vi "Client simulator.vi"() -> ()   [LabVIEW 2011]
panel:
  in  "?":bool
  in  "Port":u16=8222 min=1025 step=1
  out "FINAL FRAME":string[](array[string])
  out "CHECK SUM":u8=202 format="%01x"
  out "ANALOG PAR":u8[](array[numeric]) format="%02x"
  out "Array 2":bool[][](array[boolean])
  out "DIGITAL PAR":u8[](array[numeric]) format="%02x"
  in  "FT":string[](array[string])
  in  "stop":bool
  in  "Stop sync":string[](array[string])
  in  "Start sync":string[](array[string])
  in  "DCNT":string[](array[string])
  in  "ACNT":string[](array[string])
  in  "Digital parameters":i32(listbox)
  in  "Analog parameters":i32(listbox)
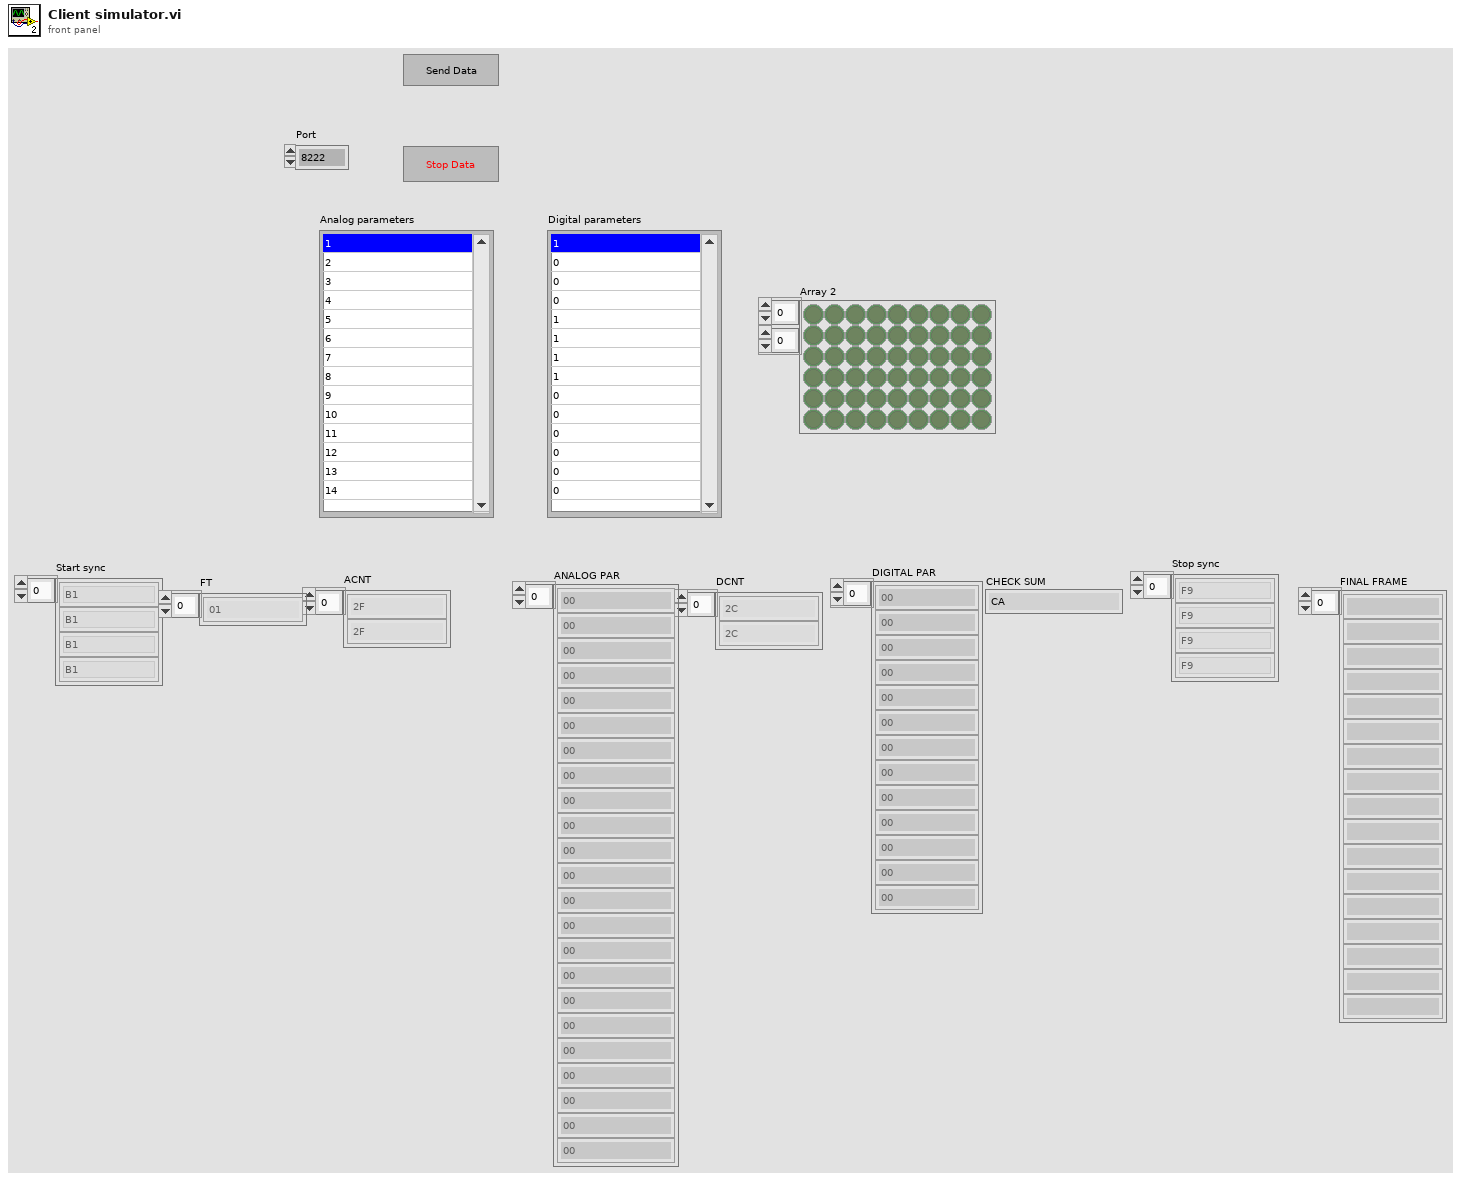
[diagram p1: front panel]
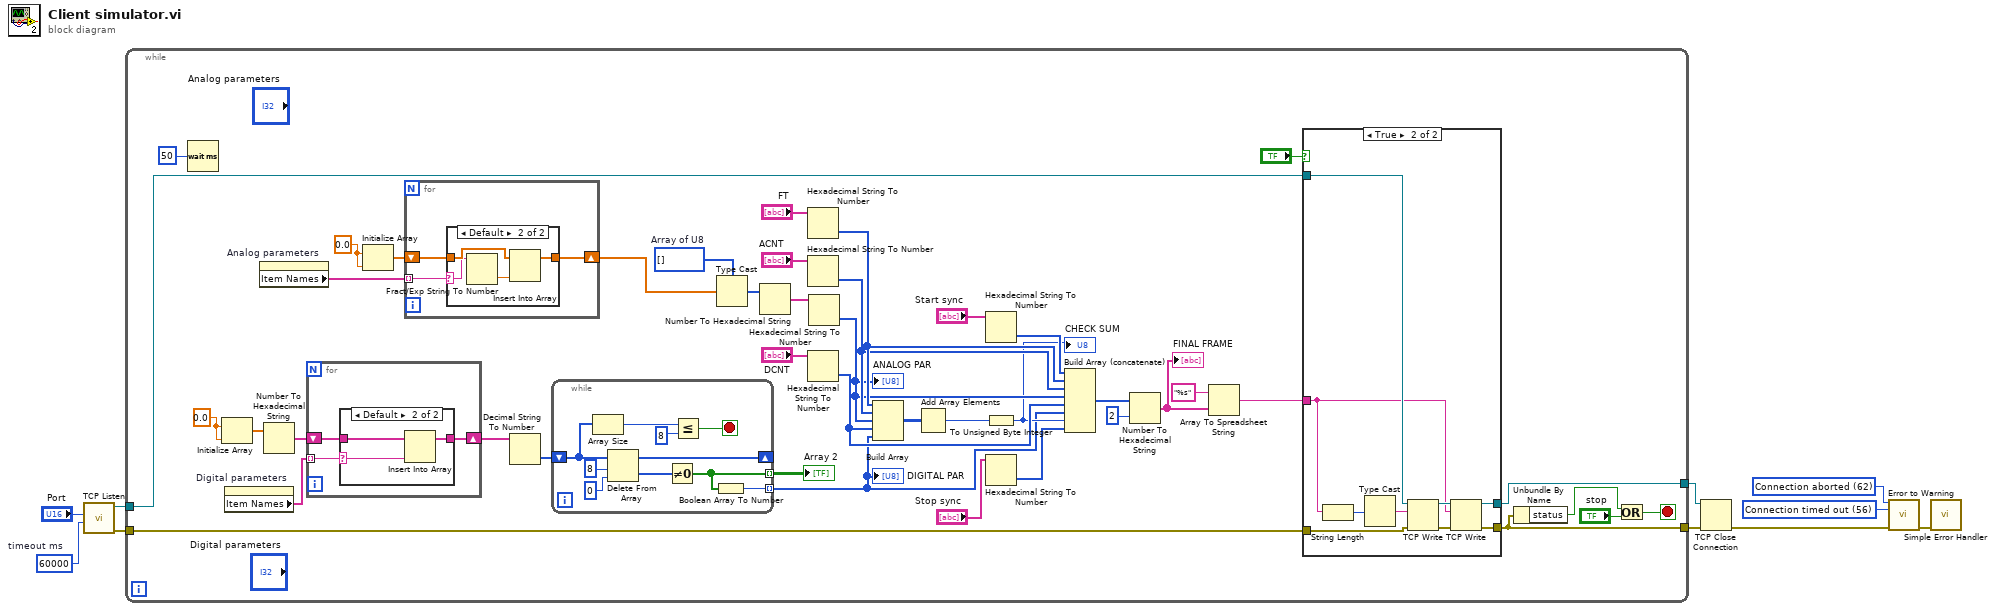
[diagram p0: block diagram]
diagram:
  w3 = 62 items=["No Error", "Argument Error", "Memory Full", "Out of Zone", "End of File", "File Already Open", "Generic File IO Error", "File Not Found", "File Permission Error", "Disk Full", "Duplicate Path", "Too Many Files Open", "Not Enabled", "Resource File Not Found", "Cannot Add Resource", "Resource Not Found", "Image Not Found", "Image Memory Error", "Pen Does Not Exist", "Config Bad Type", "Config Token Not Found", "Config Parse Error", "Config Memory Error", "Bad External Code Format", "Bad External Code Offset", "External Code Not Present", "Null Window", "Destroy Window Mixup", "Null Menu", "Print Aborted", "Bad Print Record", "Print Driver Error", "Windows Error During Print", "Memory Error During Print", "Print Dialog Error", "Generic Print Error", "Invalid Device Refnum", "Device Not Found", "Device Parameter Error", "Device Unit Error", "Can't Open Device", "Device Call Aborted", "Generic Error", "Cancelled By User", "Object ID Too Low", "Object ID Too High", "Object Not In Heap", "Unknown Heap", "Bad DefProc ID", "DefProc Not In Table", "Message Out Of Range", "Null Method", "Unknown Message", "Manager Call Not Supported", "Bad address", "Connection In progress", "Connection timed out", "Connection is already in progress", "Network attribute not supported", "Network error", "Address in use", "System out of memory", "Connection aborted", "Connection refused", "Connection is not connected", "Connection is already connected", "Connection closed", "Initialize error (interapplication manager)", "Bad occurrence", "Wait on unbound occurrence handler", "Occurrence queue overflow", "Bad path", "Semaphore not signaled", "Unrecognized type (interapplication manager)"] ("1st Error to Convert")
  w2 = 56 items=["No Error", "Argument Error", "Memory Full", "Out of Zone", "End of File", "File Already Open", "Generic File IO Error", "File Not Found", "File Permission Error", "Disk Full", "Duplicate Path", "Too Many Files Open", "Not Enabled", "Resource File Not Found", "Cannot Add Resource", "Resource Not Found", "Image Not Found", "Image Memory Error", "Pen Does Not Exist", "Config Bad Type", "Config Token Not Found", "Config Parse Error", "Config Memory Error", "Bad External Code Format", "Bad External Code Offset", "External Code Not Present", "Null Window", "Destroy Window Mixup", "Null Menu", "Print Aborted", "Bad Print Record", "Print Driver Error", "Windows Error During Print", "Memory Error During Print", "Print Dialog Error", "Generic Print Error", "Invalid Device Refnum", "Device Not Found", "Device Parameter Error", "Device Unit Error", "Can't Open Device", "Device Call Aborted", "Generic Error", "Cancelled By User", "Object ID Too Low", "Object ID Too High", "Object Not In Heap", "Unknown Heap", "Bad DefProc ID", "DefProc Not In Table", "Message Out Of Range", "Null Method", "Unknown Message", "Manager Call Not Supported", "Bad address", "Connection In progress", "Connection timed out", "Connection is already in progress", "Network attribute not supported", "Network error", "Address in use", "System out of memory", "Connection aborted", "Connection refused", "Connection is not connected", "Connection is already connected", "Connection closed", "Initialize error (interapplication manager)", "Bad occurrence", "Wait on unbound occurrence handler", "Occurrence queue overflow", "Bad path", "Semaphore not signaled", "Unrecognized type (interapplication manager)"] ("2nd Error to Convert")
  w9 = 60000  # timeout ms
  n1 = call <vilib>:"TCP Listen.vi"("timeout ms (wait forever: -1)"=w9, "port"="Port") -> ("error out"=w7:errorcluster, "connection ID"=w8:refnum<k5>)  [unwired: 5 in, 3 out]
  n2 = while {
    tunnel: w8 -> [w23]
    tunnel: w7 -> [w22]
    tunnel: [w13] -> w5
    tunnel: [w14] -> w6
    stop <- w16 stop-if-true
    w44 = sgl 0.0 ("dimension size")
    w51 = u8[] []  # Array of U8
    w53 = sgl 0.0 ("dimension size")
    n3 = Wait (ms)(milliseconds to wait=u32 50) -> ()  [unwired: 1 out]
    n4 = Initialize Array(w44, w44) -> (w46:sgl[])
    n5 = property on="Digital parameters" class="LstBox (strict)"() -> ("Item Names"=w47:string[])  [unwired: 2 in, 2 out]
    n6 = property on="Analog parameters" class="LstBox (strict)"() -> ("Item Names"=w49:string[])  [unwired: 2 in, 2 out]
    n7 = Number To Hexadecimal String(2:w46) -> (0:w45:string[])  [unwired: 1 in]
    n8 = for {
      shift-right: [w76] -> w11
      shift-left: w45 -> [w77]
      tunnel: w47 -> [w75] mode=indexing
      n9 = case shown="Default" w75 {
        selector: w75 -> [_ w79]
        tunnel: w77 -> [w78 w81]
        tunnel: [w78 w80] -> w76
        frame "" {
        }
        frame Default {
          n10 = Insert Into Array(array=w81, new element=w79) -> (w80:string[])  [unwired: 1 in]
        }
      }
    }
    n11 = Initialize Array(w53, w53) -> (w48:sgl[])
    n12 = for {
      shift-right: [w83] -> w24
      shift-left: w48 -> [w84]
      tunnel: w49 -> [w82] mode=indexing
      n13 = case shown="Default" w82 {
        selector: w82 -> [_ w87]
        tunnel: w84 -> [w85 w89]
        tunnel: [w85 w88] -> w83
        frame "" {
        }
        frame Default {
          n14 = Fract/Exp String To Number(string=w87) -> (number=w86:dbl)  [unwired: 3 in, 1 out]
          n15 = Insert Into Array(array=w89, new element=w86) -> (w88:sgl[])  [unwired: 1 in]
        }
      }
    }
    n16 = Decimal String To Number(string=w11) -> (number=w43:i32[])  [unwired: 2 in, 1 out]
    n17 = while {
      shift-right: [w68] -> _
      shift-left: w43 -> [w74]
      tunnel: [w66] -> w42 mode=indexing
      tunnel: [w65] -> w12 mode=indexing
      stop <- w71 stop-if-true
      n18 = Array Size(array=w74) -> (size(s)=w73:i32)
      n19 = Delete From Array(array=w74, length=8, index=0) -> (deleted portion=w67:i32[], array with subset deleted=w68:i32[])
      n20 = Not Equal To 0?(x=w67) -> (x != 0?=w66:bool[])
      n21 = Less Or Equal?(x=w73, y=8) -> (x <= y?=w71:bool)
      n22 = Boolean Array To Number(Boolean array=w66) -> (number=w65:u32)
    }
    "Array 2" <- w42
    "DIGITAL PAR" <- w12
    n23 = Type Cast(type=w51, x=w24) -> (*(type *) &x=w50:u8[])
    n24 = Number To Hexadecimal String(2:w50) -> (0:w41:string[])  [unwired: 1 in]
    n25 = Hexadecimal String To Number(string="FT") -> (number=w33:u32[])  [unwired: 2 in, 1 out]
    n26 = Hexadecimal String To Number(string="ACNT") -> (number=w32:u32[])  [unwired: 2 in, 1 out]
    n27 = Hexadecimal String To Number(string="DCNT") -> (number=w30:u32[])  [unwired: 2 in, 1 out]
    n28 = Hexadecimal String To Number(string=w41) -> (number=w31:u32[])  [unwired: 2 in, 1 out]
    "ANALOG PAR" <- w31
    n29 = Build Array(w33, w32, w31, w30, w12) -> (w37:u32[][])
    n30 = Add Array Elements(numeric array=w37) -> (sum=w27:u32)
    n31 = Hexadecimal String To Number(string="Start sync") -> (number=w34:u32[])  [unwired: 2 in, 1 out]
    n32 = To Unsigned Byte Integer(number=w27) -> (unsigned 8bit integer=w26:u8)
    "CHECK SUM" <- w26
    n33 = Hexadecimal String To Number(string="Stop sync") -> (number=w29:u32[])  [unwired: 2 in, 1 out]
    n34 = Build Array (concatenate)(w34, w33, w32, w31, w30, w12, w26, w29) -> (w28:u32[])
    n35 = Number To Hexadecimal String(1:i16 2 ("width (-)"), 2:w28) -> (0:w21:string[])
    "FINAL FRAME" <- w21
    n36 = Array To Spreadsheet String(array=w21, 3:"%s" ("format string")) -> (spreadsheet string=w19:string)  [unwired: 1 in]
    n37 = case shown="True" "?" {
      tunnel: w23 -> [w55 w64]
      tunnel: w22 -> [w54 w63]
      tunnel: w19 -> [_ w60]
      tunnel: [w55 w57] -> w14
      tunnel: [w54 w56] -> w13
      frame False {
      }
      frame True {
        n38 = String Length(string=w60) -> (length=w59:i32)
        n39 = Type Cast(x=w59) -> (*(type *) &x=w58:string)  [unwired: 1 in]
        n40 = TCP Write(connection ID=w64, data in=w58, error in (no error)=w63) -> (connection ID out=w62:refnum<k5>, error out=w61:errorcluster)  [unwired: 1 in, 1 out]
        n41 = TCP Write(connection ID=w62, data in=w60, error in (no error)=w61) -> (connection ID out=w57:refnum<k5>, error out=w56:errorcluster)  [unwired: 1 in, 1 out]
      }
    }
    n42 = Unbundle By Name(w13) -> ("status"=w17:bool)
    n43 = Or(x=w17, y="stop") -> (x .or. y?=w16:bool)
  }
  n44 = TCP Close Connection(connection ID=w6, error in (no error)=w5) -> (error out=w4:errorcluster)  [unwired: 1 in, 1 out]
  n45 = call <vilib>:"Error to Warning.vi"("1st Error to Convert"=w3, "2nd Error to Convert"=w2, "error in"=w4) -> ("warning out"=w1:errorcluster)  [unwired: 12 in]
  n46 = call <vilib>:"Simple Error Handler.vi"("error in (no error)"=w1) -> ()  [unwired: 4 in, 5 out]
